vi "Two Pixels to Segment.vi"(8 "Error In":errorcluster, 9 "Pixel 2":cluster{"X":i32, "Y":i32}, 11 "Pixel 1":cluster{"X":i32, "Y":i32}) -> (0 "Error Out":errorcluster, 3 "Segment 1-2":cluster{"Array":i32[]})   [LabVIEW 2021, in "Image.lvlib"]
uses:
  Image.lvlib
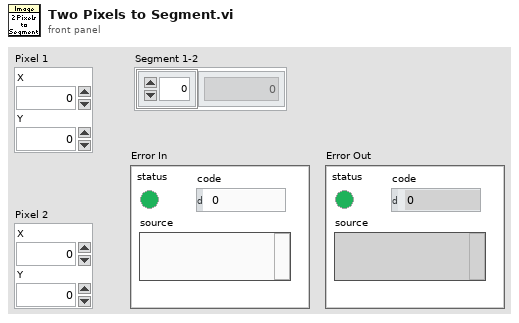
[diagram p1: front panel]
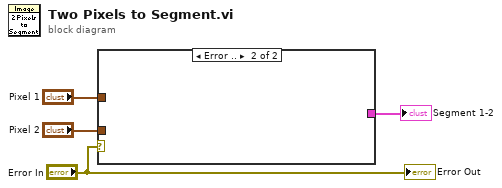
[diagram p0: block diagram]
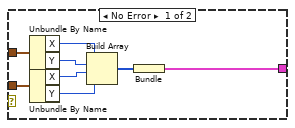
[diagram p2: hidden frame]
diagram:
  n1 = case shown="Error .." "Error In" {
    tunnel: [w12 _] -> w4
    tunnel: "Pixel 2" -> [w6 _]
    tunnel: "Pixel 1" -> [w5 _]
    frame No Error {
      n2 = Unbundle By Name(w5) -> ("X"=w7:i32, "Y"=w9:i32)
      n3 = Unbundle By Name(w6) -> ("X"=w10:i32, "Y"=w8:i32)
      n4 = Build Array(w7, w9, w10, w8) -> (w11:i32[])
      n5 = Bundle(w11) -> (w12:cluster{i32[]})  [unwired: 1 in]
    }
    frame Error {
    }
  }
  "Segment 1-2" <- w4
  "Error Out" <- "Error In"
